vi "fftw_test_sine.vi"() -> ()   [LabVIEW 2020]
uses:
  Window Type.ctl
  FFTWDLL.lvlib
panel:
  in  "window type":T1
  in  "Log y-scale?":bool
  out "wave spectrum":dbl[](graph)
  in  "stop":bool
  in  "samples":i32=10000
  out "wave in":dbl[](graph)
  in  "Coherent?":bool
  in  "amplitude [-]":dbl(slide) min=0.0 max=1.0 scale=0.0..1.0
  in  "frequency [-]":dbl(slide) min=0.0 max=0.5 scale=0.0..0.5
  out "error out":errorcluster
  in  "error in (no error)":errorcluster
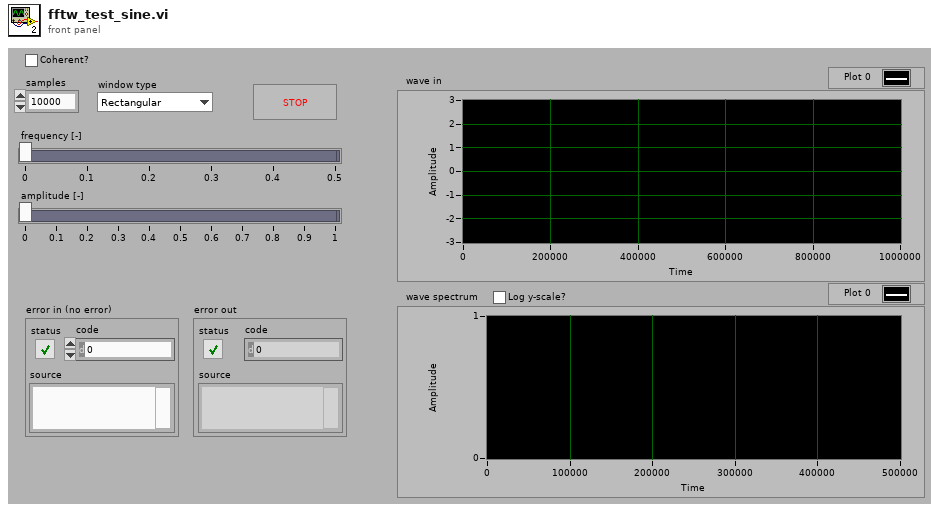
[diagram p1: front panel]
types:
  T1 = typedef "Window Type.ctl" = enum16{"Rectangular", "Hanning", "Blackman-Harris"}
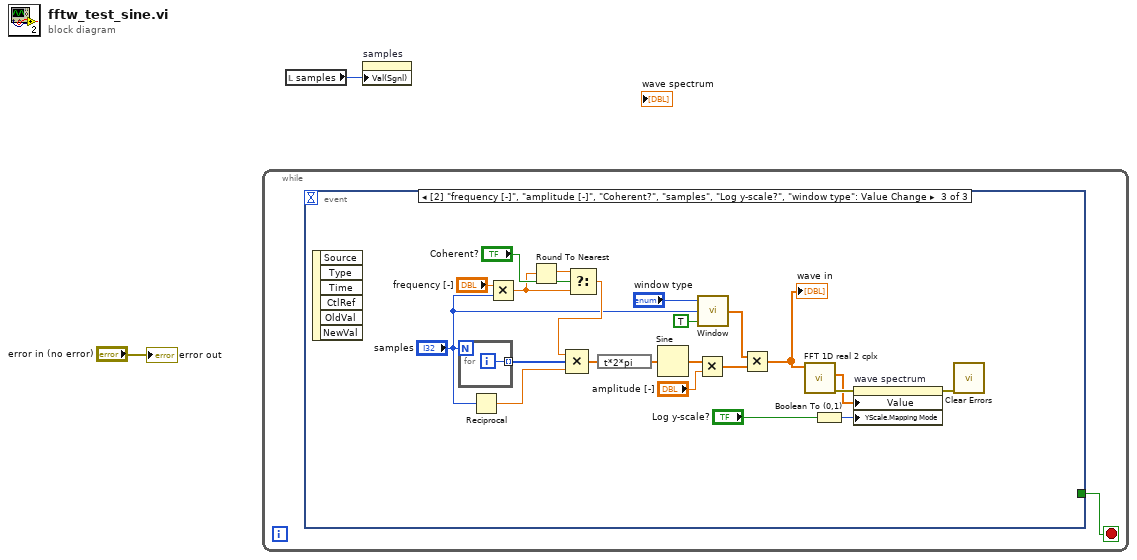
[diagram p0: block diagram]
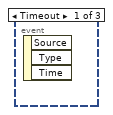
[diagram p2: hidden frame]
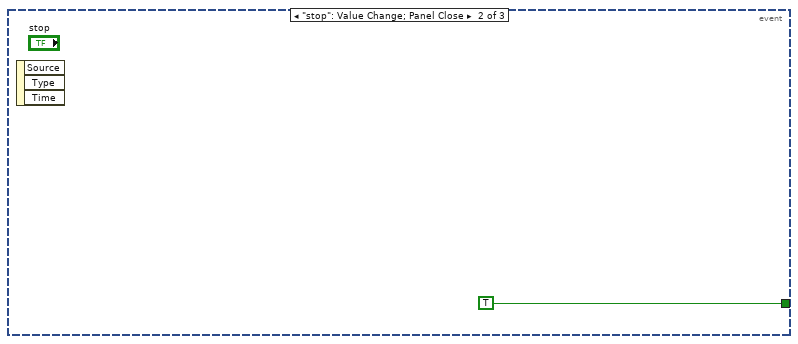
[diagram p3: hidden frame]
diagram:
  n1 = while {
    stop <- w3 stop-if-true
    n2 = event shown="[2] \"frequency [-]\", \"amplitude [-]\", \"Coherent?\", \"samples\", \"Log y-scale?\", \"window type\": Value Change" {
      selector: _ -> [_ _ _]
      dyn-events: _ -> [_ _ _]
      timeout: _ -> [_ _ _]
      tunnel: [_ TRUE _] -> w3
      event Timeout {
        n3 = event-data() -> ()  [unwired: 1 in, 3 out]
      }
      event "stop": Value Change; Panel Close {
        n4 = event-data() -> ()  [unwired: 1 in, 3 out]
      }
      event "frequency [-]", "amplitude [-]", "Coherent?", "samples", "Log y-scale?": Value Change {
        n5 = event-data() -> ()  [unwired: 1 in, 6 out]
        n6 = for {
          N: "samples" -> [_]
          tunnel: [w27] -> w24 mode=indexing
          i -> [w27]
        }
        n7 = Reciprocal(x="samples") -> (1/x=w23:dbl)
        n8 = Multiply(x="frequency [-]", y="samples") -> (x*y=w19:dbl)
        n9 = Round To Nearest(number=w19) -> (nearest integer value=w20:dbl)
        n10 = Select(t=w20, s="Coherent?", f=w19) -> (s? t:f=w18:dbl)
        n11 = Compound Arithmetic op=MULTIPLY(w18, w24, w23) -> (w26:dbl[])
        n12 = expression code="t*2*pi"(w26) -> (w25:dbl[])
        n13 = Sine(x=w25) -> (sin(x)=w17:dbl[])
        n14 = Multiply(x=w17, y="amplitude [-]") -> (x*y=w7:dbl[])
        n15 = call "Window.vi"("Normalize? (False)"=TRUE, "N"="samples", "window type"="window type") -> ("window"=w6:dbl[])
        n16 = Multiply(x=w6, y=w7) -> (x*y=w5:dbl[])
        "wave in" <- w5
        n17 = call "FFT 1D real 2 cplx.vi"("y"=w5) -> ("error out"=w15:errorcluster, "amp(Y)"=w14:dbl[])  [unwired: 7 in, 2 out]
        n18 = Boolean To (0,1)(Boolean="Log y-scale?") -> (0, 1=w11:i16)
        n19 = property on="wave spectrum" class="WFGraph (strict)"(error in=w15, "Value"=w14, "YScale.Mapping Mode"=w11) -> (error out=w13:errorcluster)  [unwired: 1 in, 1 out]
        n20 = call <vilib>:"Clear Errors.vi"("error in (no error)"=w13) -> ()  [unwired: 5 in, 2 out]
      }
    }
  }
  n21 = local read "samples"() -> (w1:i32)
  n22 = property on="samples" class="DigNum (strict)"("Val(Sgnl)"=w1) -> ()  [unwired: 2 in, 2 out]
  "error out" <- "error in (no error)"
